vi "Create CONNACK Packet.vi"(5 "CONNACK type":refnum<class "CONNACK.lvclass">, 8 "error in (no error)":errorcluster, 10 "Return Code":T1, 11 "Session Present":bool) -> (0 "error out":errorcluster, 3 "CONNACK":refnum<class "CONNACK.lvclass">)   [LabVIEW 2013, in "CONNACK.lvclass"]
uses:
  CONNACK.lvclass
  Connect Return Code -- enum.ctl
  ControlPacket/ControlPacket.lvclass/ControlPacket.ctl
  ControlPacket/ControlPacket.lvclass
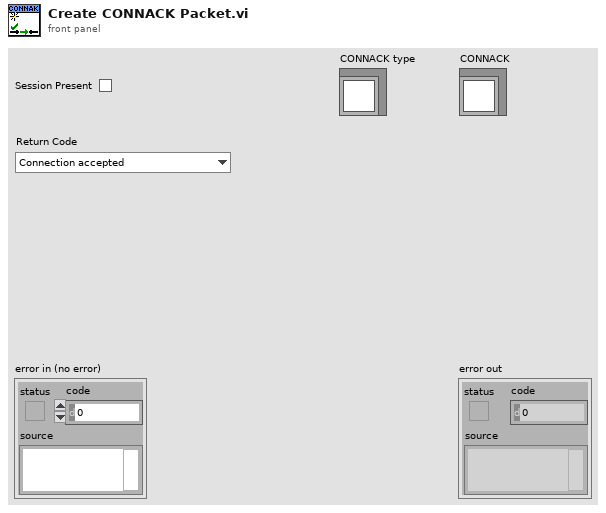
[diagram p1: front panel]
types:
  T1 = typedef "CONNACK.lvclass/Connect Return Code -- enum.ctl" = enum16{"Connection accepted", "Unacceptable protocol version", "Identifier Rejected", "Server Unavailable", "Bad Username or Password", "Not Authorized"}
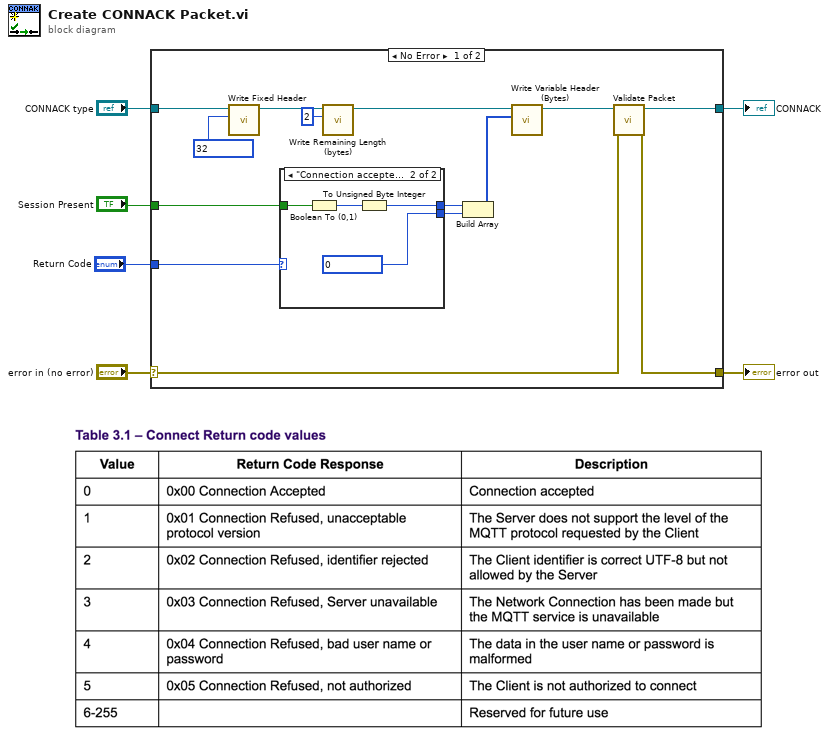
[diagram p0: block diagram]
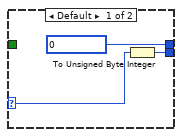
[diagram p2: hidden frame]
diagram:
  n1 = case shown="No Error" "error in (no error)" {
    selector: "error in (no error)" -> [w13 w29]
    tunnel: [w12 w29] -> w5
    tunnel: [w14 w28] -> w3
    tunnel: "CONNACK type" -> [w19 w28]
    tunnel: "Session Present" -> [w10 _]
    tunnel: "Return Code" -> [w11 _]
    frame No Error {
      n2 = call "Write Fixed Header.vi"("Fixed Header"=u8 32, "ControlPacket in"=w19) -> ("ControlPacket out"=w9:refnum<class "CONNACK.lvclass">)  [unwired: 9 in]
      n3 = case shown="\"Connection accepted\"" w11 {
        selector: w11 -> [w21 _]
        tunnel: [u8 0 w24] -> w16
        tunnel: [w23 u8 0] -> w15
        tunnel: w10 -> [_ w26]
        frame Default {
          n4 = To Unsigned Byte Integer(number=w21) -> (unsigned 8bit integer=w23:u8)
        }
        frame "Connection accepted" {
          n5 = Boolean To (0,1)(Boolean=w26) -> (0, 1=w25:i16)
          n6 = To Unsigned Byte Integer(number=w25) -> (unsigned 8bit integer=w24:u8)
        }
      }
      n7 = call "Write Remaining Length (bytes).vi"("Remaining Length (bytes)"=u32 2, "ControlPacket in"=w9) -> ("ControlPacket out"=w8:refnum<class "CONNACK.lvclass">)  [unwired: 9 in]
      n8 = Build Array(w16, w15) -> (w18:u8[])
      n9 = call "Write Variable Header (Bytes).vi"("Variable Header (Bytes)"=w18, "ControlPacket in"=w8) -> ("ControlPacket out"=w17:refnum<class "CONNACK.lvclass">)  [unwired: 9 in]
      n10 = call "Validate Packet.vi"("error in (no error)"=w13, "ControlPacket in"=w17) -> ("error out"=w12:errorcluster, "ControlPacket out"=w14:refnum<class "CONNACK.lvclass">)  [unwired: 8 in]
    }
    frame Error {
    }
  }
  "error out" <- w5
  "CONNACK" <- w3
